vi "IR Field Positioning.vi"(8 "Right":bool, 9 "Left":bool, 11 "Encoder data":T1 {"Omni"."Ticks" format="%#.6g"; "Right"."Ticks" format="%#.6g"; "Left"."Ticks" format="%#.6g"}) -> ()   [LabVIEW 2013]
uses:
  Encoder Data.ctl
  Single Encoder Data.ctl
  Common Code/Change Detect Boolean.vi
  Robot Global Data.vi
  <vilib>/Rock Robotics/WPI/Gyro/WPI_GyroRefNum Registry Get.vi
  <vilib>/Rock Robotics/WPI/Gyro/WPI_GyroGetAngle.vi
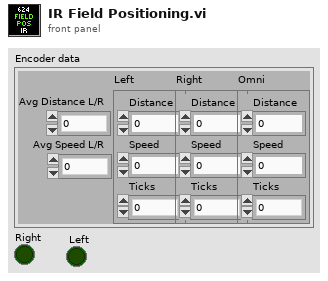
[diagram p1: front panel]
types:
  T1 = typedef "Encoder Data.ctl" = cluster{"Avg Distance L/R":dbl, "Avg Speed L/R":dbl, "Left":T2, "Right":T2, "Omni":T2}
  T2 = typedef "Single Encoder Data.ctl" = cluster{"Distance":dbl, "Speed":dbl, "Ticks":dbl}
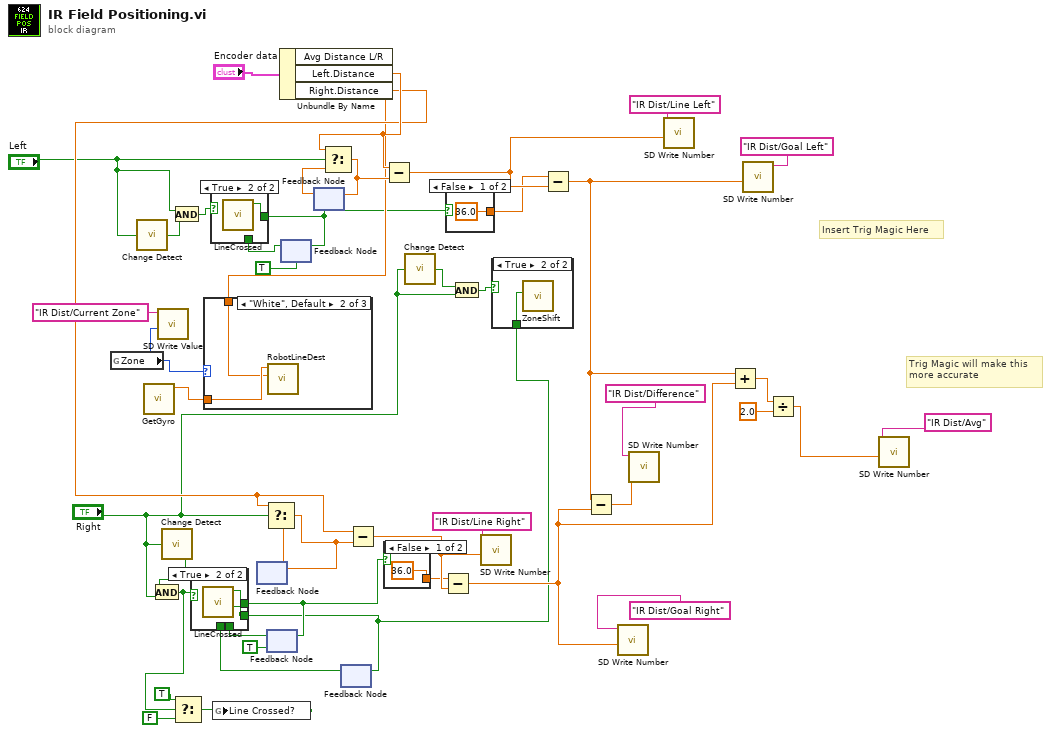
[diagram p0: block diagram]
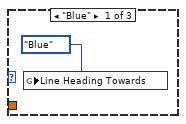
[diagram p5: hidden frame]
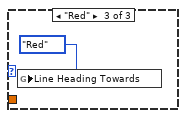
[diagram p6: hidden frame]
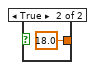
[diagram p7: hidden frame]
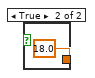
[diagram p8: hidden frame]
diagram:
  # "Trig Magic will make this\nmore accurate"
  # "Insert Trig Magic Here"
  n1 = global read "Robot Global Data.vi" "Zone"() -> (w22:enum16{"Blue", "White", "Red"})
  n2 = call-poly "Change Detect.vi"("In"="Left") -> ("Changed?"=w15:bool)
  n3 = call "GetGyro.vi"() -> ("Angle"=w30:dbl)  [unwired: 9 in, 2 out]
  n4 = call-poly <vilib>:"SD Write Value.vi"("Numeric"=w22, "Name"="IR Dist/Current Zone") -> ()  [unwired: 8 in, 2 out]
  n5 = call-poly "Change Detect.vi"("In"="Right") -> ("Changed?"=w16:bool)
  n6 = And(x=w16, y="Right") -> (x .and. y?=w9:bool)
  n7 = And(x="Left", y=w15) -> (x .and. y?=w14:bool)
  n8 = Select(t=TRUE ("s"), s=w9, f=FALSE) -> (s? t:f=w6:bool)
  n9 = global write "Robot Global Data.vi" "Line Crossed?"(w6) -> ()
  n10 = feedback #1() -> (w43:dbl)  [unwired: 1 in]
  n11 = feedback #2(TRUE ("Onside")) -> (w25:bool)
  n12 = Unbundle By Name("Encoder data") -> ("Avg Distance L/R"=w29:dbl, "Left.Distance"=w45:dbl, "Right.Distance"=w31:dbl)
  n13 = case shown="\"White\", Default" w22 {
    tunnel: w30 -> [_ w49 _]
    tunnel: w29 -> [_ w48 _]
    frame "Blue" {
      n14 = global write "Robot Global Data.vi" "Line Heading Towards"(enum16{"Red", "Blue"}."Blue" ("Line Heading Towards")) -> ()
    }
    frame "White", Default {
      n15 = call "RobotLineDest.vi"("Average Distance"=w48, "Angle"=w49) -> ()  [unwired: 10 in]
    }
    frame "Red" {
      n16 = global write "Robot Global Data.vi" "Line Heading Towards"(enum16{"Red", "Blue"}."Red" ("Line Heading Towards")) -> ()
    }
  }
  n17 = Select(t=w31, s="Right", f=w43) -> (s? t:f=w46:dbl)
  n18 = feedback-in #1(w46) -> ()
  n19 = feedback #3(TRUE ("Onside")) -> (w27:bool)
  n20 = case shown="True" w14 {
    tunnel: [w51 w52] -> w28
    tunnel: w27 -> [w51 _]
    frame False {
    }
    frame True {
      n21 = call "LineCrossed.vi"() -> ("Onside"=w52:bool)  [unwired: 10 in, 1 out]
    }
  }
  n22 = feedback-in #3(w28) -> ()
  n23 = feedback #4() -> (w44:dbl)  [unwired: 1 in]
  n24 = Select(t=w45, s="Left", f=w44) -> (s? t:f=w41:dbl)
  n25 = feedback-in #4(w41) -> ()
  n26 = feedback #5() -> (w13:bool)  [unwired: 1 in]
  n27 = case shown="True" w9 {
    tunnel: [w54 w56] -> w26
    tunnel: w25 -> [w54 _]
    tunnel: [w53 w55] -> w12
    tunnel: w13 -> [w53 _]
    frame False {
    }
    frame True {
      n28 = call "LineCrossed.vi"() -> ("LineDir"=w55:bool, "Onside"=w56:bool)  [unwired: 10 in]
    }
  }
  n29 = feedback-in #2(w26) -> ()
  n30 = feedback-in #5(w12) -> ()
  n31 = Subtract(x=w31, y=w46) -> (x-y=w42:dbl)
  n32 = Subtract(x=w45, y=w41) -> (x-y=w40:dbl)
  n33 = case shown="False" w26 {
    tunnel: [36.0 ("x") 18.0 ("x")] -> w37
    frame False {
    }
    frame True {
    }
  }
  n34 = call-poly "Change Detect.vi"("In"="Right") -> ("Changed?"=w10:bool)
  n35 = Subtract(x=w37, y=w42) -> (x-y=w18:dbl)
  n36 = case shown="False" w28 {
    tunnel: [36.0 ("abs(x)") 18.0 ("abs(x)")] -> w33
    frame False {
    }
    frame True {
    }
  }
  n37 = And(x=w10, y="Right") -> (x .and. y?=w11:bool)
  n38 = call <vilib>:"SD Write Number.vi"("Numeric"=w42, "Name"="IR Dist/Line Right") -> ()  [unwired: 8 in, 2 out]
  n39 = case shown="True" w11 {
    tunnel: w12 -> [_ w61]
    frame False {
    }
    frame True {
      n40 = call "ZoneShift.vi"("LineDir"=w61) -> ()  [unwired: 11 in]
    }
  }
  n41 = Subtract(x=w33, y=w40) -> (x-y=w17:dbl)
  n42 = Subtract(x=w17, y=w18) -> (x-y=w38:dbl)
  n43 = call <vilib>:"SD Write Number.vi"("Numeric"=w18, "Name"="IR Dist/Goal Right") -> ()  [unwired: 8 in, 2 out]
  n44 = call <vilib>:"SD Write Number.vi"("Numeric"=w38, "Name"="IR Dist/Difference") -> ()  [unwired: 8 in, 2 out]
  n45 = call <vilib>:"SD Write Number.vi"("Numeric"=w40, "Name"="IR Dist/Line Left") -> ()  [unwired: 8 in, 2 out]
  n46 = Add(x=w17, y=w18) -> (x+y=w20:dbl)
  n47 = call <vilib>:"SD Write Number.vi"("Numeric"=w17, "Name"="IR Dist/Goal Left") -> ()  [unwired: 8 in, 2 out]
  n48 = Divide(x=w20, y=2.0) -> (x/y=w4:dbl)
  n49 = call <vilib>:"SD Write Number.vi"("Numeric"=w4, "Name"="IR Dist/Avg") -> ()  [unwired: 8 in, 2 out]
